vi "Waveform.vi"() -> ()   [LabVIEW 2016]
uses:
  controls/ScanWaveform.ctl
  controls/Enum.ctl
  <vilib>/Utility/error.llb/Error Cluster From Error Code.vi
  <vilib>/rvi/errors/niLvFpgaAdjustHostInterfaceError.vi
  <vilib>/rvi/interface/nirviReadWriteControl/nirviReadWriteControl.xnode
  controls/FPGAVIreferenceTypeDefScanEngine.ctl
  FPGA Bitfiles/qnmController797_usbRIO_controllerFPGAmu_11012018-14h.lvbitx
  NiFpgaLv.dll
panel:
  in  "scanWaveFormCtl":T2={"slowWavePts"=1024, "fastWavePts"=1024, "slowWaveType"=enum."Triangle", "fastWaveType"=enum."Rounded", "slowRoundPts"=8, "fastRoundPts"=32, "Update Parameters"=FALSE, "Correct Hysteresis"=FALSE, "UpdateFPGA"=FALSE, "Update Graph"=FALSE, "Hysteresis comp?"=FALSE}
  out "Waveforms":waveform(dbl)[](graph)
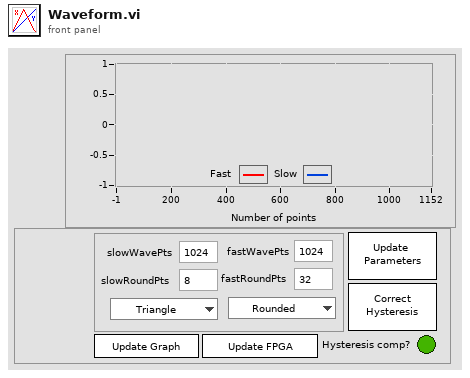
[diagram p1: front panel]
types:
  T1 = typedef "ScanWaveform.ctl" = enum16{"Sine", "Triangle", "Rounded"}
  T2 = cluster{"slowWavePts":u16, "fastWavePts":u16, "slowWaveType":T1, "fastWaveType":T1, "slowRoundPts":u16, "fastRoundPts":u16, "Update Parameters":bool, "Correct Hysteresis":bool, "UpdateFPGA":bool, "Update Graph":bool, "Hysteresis comp?":bool}
  T3 = enum16{"Init", "Update.Parameters", "Correct.Hysteresis", "Send.Waveform", "Refresh.Graph", "WaitForEvents", "Close"}
  T4 = typedef "Enum.ctl" = enum16{"Init", "Read", "Write"}
  T5 = cluster{"write":bool, "index":u16, "data":fxp<+/-,18,5>}
  T6 = cluster{"CorrectionToFGV":bool, "PolynomCoeff":dbl[], "CorrectionToFPGA":bool}
  T7 = typedef "FPGAVIreferenceTypeDefScanEngine.ctl" = refnum<k20>
  T8 = cluster{"slowWavePts":u16, "fastWavePts":u16, "slowWaveType":T1, "fastWaveType":T1, "slowRoundPts":u16, "fastRoundPts":u16, "singleDirectionScan":bool}
  T9 = cluster{"startFwd":u16, "endFwd":u16, "startBwd":u16, "endBwd":u16, "disableBlanking":bool, "useFineCounter":bool}
  T10 = cluster{"outputRate":u16, "fastDecFactor":u16, "outWaveSizeFast":u16, "pplUpsampling":u16, "numLines":u16, "se.p.fastInvDec":fxp<+,22,0>, "se.p.slowUpStep":fxp<+,28,0>, "se.p.outWaveSizeSlow":u16, "blankingMax":u32, "se.p.fastBlanking":cluster{"startFwd":u32, "endFwd":u32, "startBwd":u32, "endBwd":u32, "disableBlanking":bool, "useCoarseCounter":bool}}
  T11 = cluster{"Waveform Shape Fast In":dbl[], "Waveform Shape Slow In":dbl[]}
  T12 = cluster{"se.p.enable":bool, "se.p.singleDirection":bool, "se.p.haltScan":bool, "se.mot.p.start":bool}
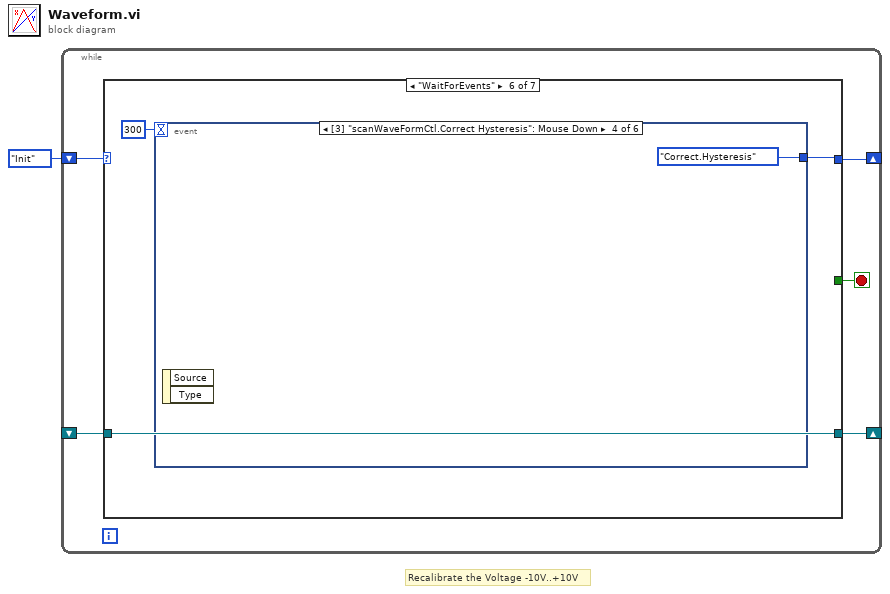
[diagram p0: block diagram]
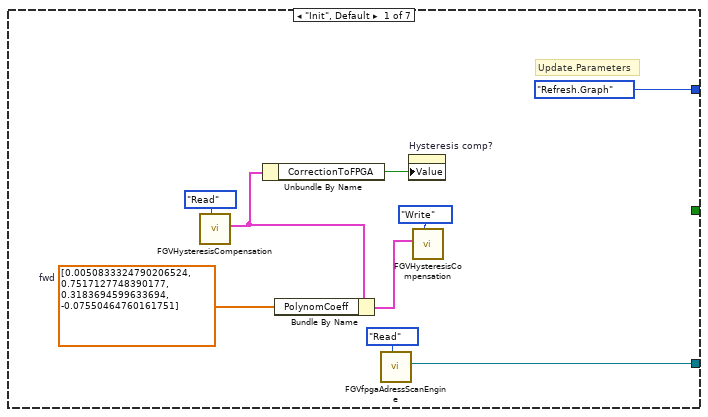
[diagram p2: hidden frame]
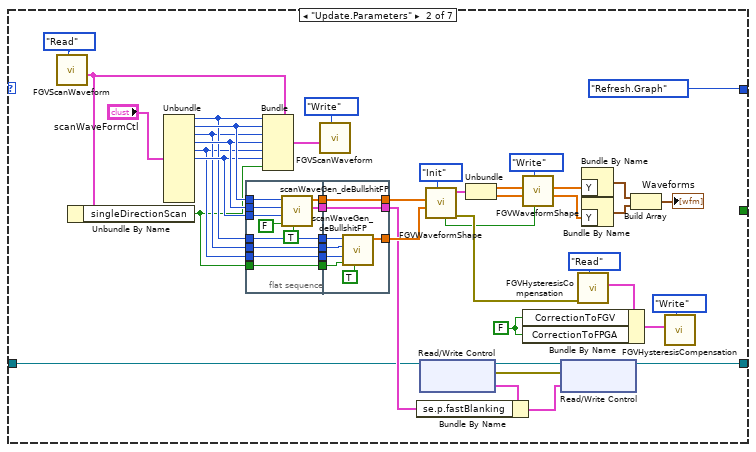
[diagram p3: hidden frame]
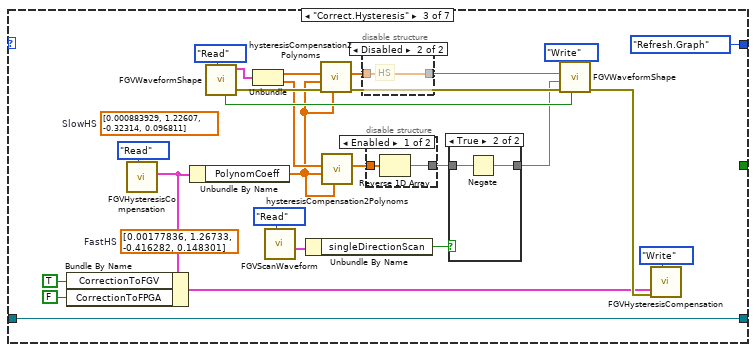
[diagram p4: hidden frame]
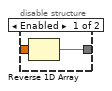
[diagram p5: hidden frame]
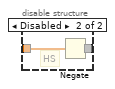
[diagram p6: hidden frame]
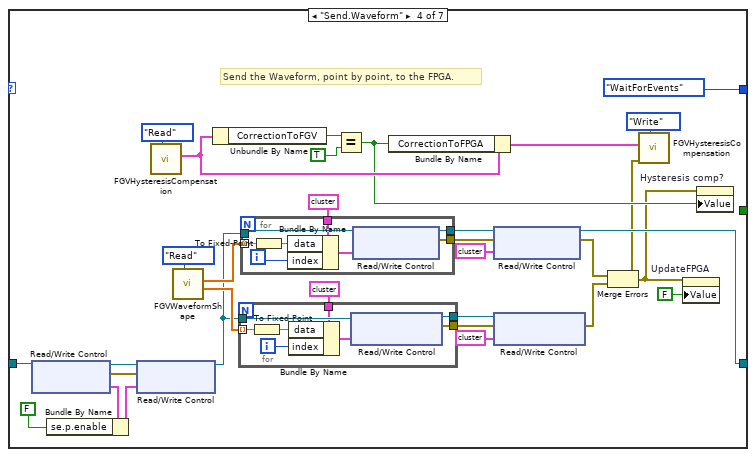
[diagram p8: hidden frame]
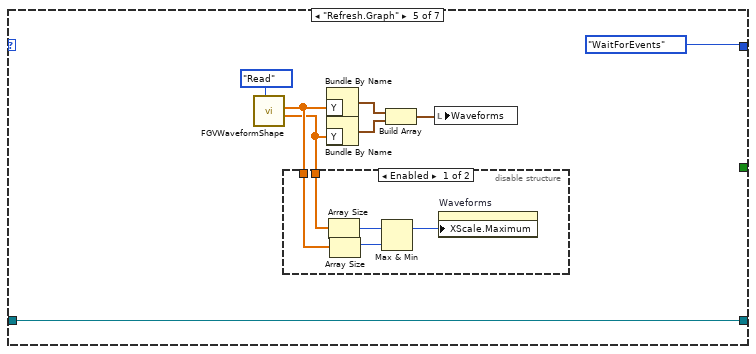
[diagram p9: hidden frame]
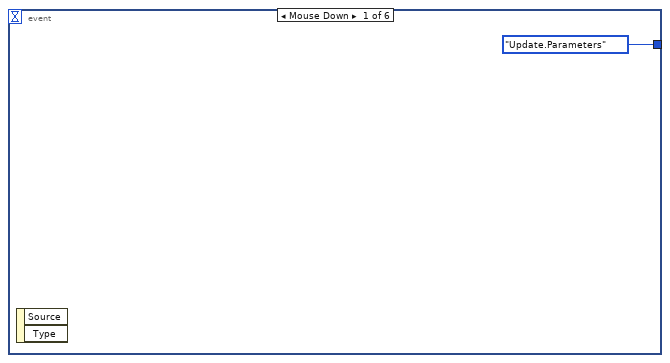
[diagram p11: hidden frame]
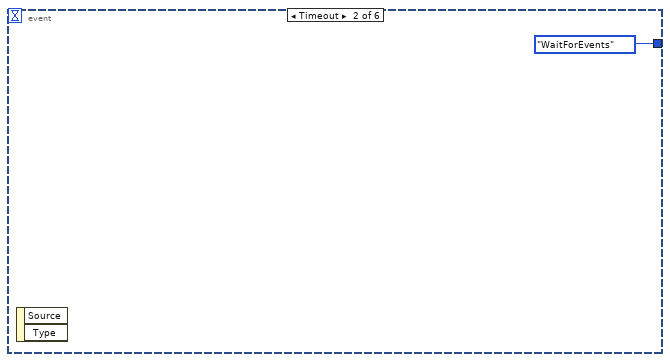
[diagram p12: hidden frame]
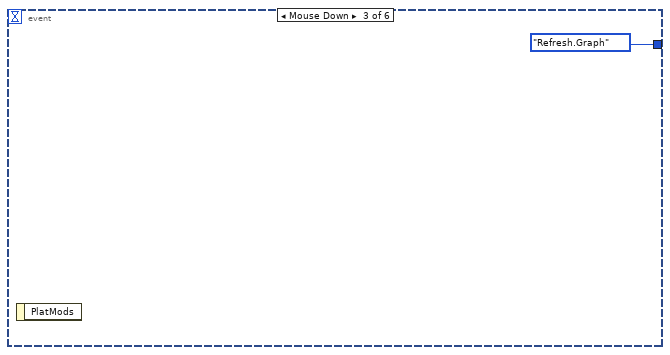
[diagram p13: hidden frame]
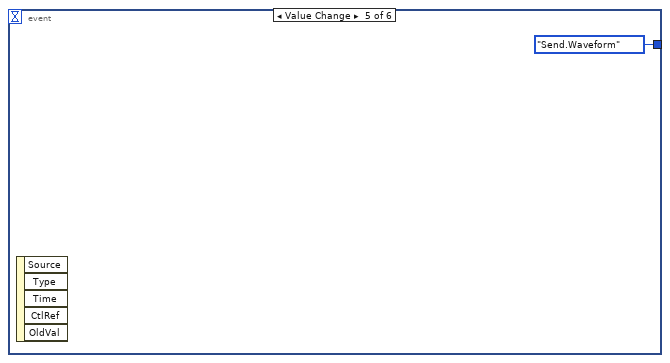
[diagram p14: hidden frame]
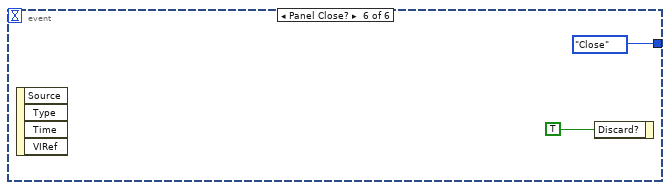
[diagram p15: hidden frame]
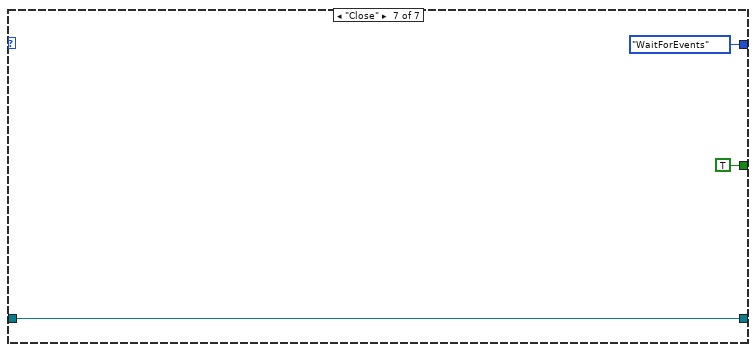
[diagram p16: hidden frame]
diagram:
  # "Recalibrate the Voltage -10V..+10V"
  n1 = while {
    shift-right: [w4] -> _
    shift-left: T3."Init" -> [w5]
    shift-right: [w3] -> _
    shift-left: _ -> [w2]
    stop <- w6 stop-if-true
    n2 = case shown="\"WaitForEvents\"" w5 {
      tunnel: [_ _ _ _ _ _ TRUE ("Discard?")] -> w6
      tunnel: [T3."Refresh.Graph" T3."Refresh.Graph" T3."Refresh.Graph" T3."WaitForEvents" T3."WaitForEvents" w177 T3."WaitForEvents"] -> w4
      tunnel: [w13 w32 w91 w126 w164 w176 w185] -> w3
      tunnel: w2 -> [_ w33 w91 w127 w164 w176 w185]
      frame "Init", Default {
        w7 = dbl[] [0.0050833324790206524, 0.7517127748390177, 0.3183694599633694, -0.07550464760161751]  # fwd
        # "Update.Parameters"
        n3 = call "FGVHysteresisCompensation.vi"("Enum"=Enum."Read") -> ("HysteresisOut"=w9:T6)  [unwired: 9 in, 1 out]
        n4 = Unbundle By Name(w9) -> ("CorrectionToFPGA"=w8:bool)
        n5 = Bundle By Name(cluster=w9, "PolynomCoeff"=w7) -> (w10:T6)
        n6 = call "FGVfpgaAdressScanEngine.vi"("Enum"=Enum."Read") -> ("FPGA.SEout"=w13:T7)  [unwired: 6 in, 4 out]
        n7 = property on="Hysteresis comp?" class="Bool (strict)"("Value"=w8) -> ()  [unwired: 2 in, 2 out]
        n8 = call "FGVHysteresisCompensation.vi"("Enum"=Enum."Write", "HysteresisIn"=w10) -> ()  [unwired: 8 in, 2 out]
      }
      frame "Update.Parameters" {
        w26 = FALSE ("Correction?")
        n9 = call "FGVScanWaveform.vi"("Enum"=Enum."Read") -> ("scanWaveFormCtl Out"=w45:T8)  [unwired: 9 in, 1 out]
        n10 = Unbundle By Name(w45) -> ("singleDirectionScan"=w38:bool)
        n11 = Unbundle("scanWaveFormCtl") -> ("slowWavePts"=w41:u16, "fastWavePts"=w44:u16, "slowWaveType"=w40:T1, "fastWaveType"=w43:T1, "slowRoundPts"=w39:u16, "fastRoundPts"=w42:u16)  [unwired: 5 out]
        n12 = flat-sequence {
          tunnel: w44 -> [w70]
          tunnel: w43 -> [w69]
          tunnel: w42 -> [w68]
          tunnel: [w66] -> w59
          tunnel: w41 -> [w66]
          tunnel: w40 -> [w65]
          tunnel: [w65] -> w58
          tunnel: [w64] -> w57
          tunnel: w39 -> [w64]
          tunnel: w38 -> [w63]
          tunnel: [w63] -> w56
          tunnel: [w62] -> w55
          tunnel: [w61] -> w54
          tunnel: w59 -> [w73]
          tunnel: w58 -> [w78]
          tunnel: w57 -> [w77]
          tunnel: w56 -> [w76]
          tunnel: w55 -> [w75]
          tunnel: [w75] -> w37
          tunnel: [w74] -> w36
          tunnel: w54 -> [w72]
          tunnel: [w72] -> w35
          frame #0 {
            n13 = call "scanWaveGen_deBullshitFP.vi"("overScanBlanking"=TRUE, "singleDirScan"=FALSE, "numRoundingPts"=w68, "scanWaveForm"=w69, "numPts"=w70) -> ("blankingParams"=w61:T9, "outWave"=w62:dbl[])  [unwired: 5 in]
          }
          frame #1 {
            n14 = call "scanWaveGen_deBullshitFP.vi"("overScanBlanking"=TRUE, "singleDirScan"=w76, "numRoundingPts"=w77, "scanWaveForm"=w78, "numPts"=w73) -> ("outWave"=w74:dbl[])  [unwired: 5 in, 1 out]
          }
        }
        n15 = Bundle(cluster=w45, "slowWavePts"=w41, "fastWavePts"=w44, "slowWaveType"=w40, "fastWaveType"=w43, "slowRoundPts"=w39, "fastRoundPts"=w42, "singleDirectionScan"=w38) -> (w47:T8)
        n16 = call "FGVScanWaveform.vi"("Enum"=Enum."Write", "scanWaveFormCtl In"=w47) -> ()  [unwired: 8 in, 2 out]
        n17 = xnode "Read/Write Control"("FPGA VI Reference In"=w33) -> ("error out"=w24:errorcluster, "se.p.clocks"=w23:T10)  [unwired: 1 in, 1 out]
        n18 = Bundle By Name(cluster=w23, "se.p.fastBlanking"=w35) -> (w22:T10)
        n19 = call "FGVWaveformShape.vi"("Enum"=Enum."Init", "Waveform Shape Slow In"=w36, "Waveform Shape Fast In"=w37) -> ("error out"=w25:errorcluster, "WaveformInit"=w31:T11, "Framing up? (down: f)"=w16:bool)  [unwired: 4 in, 2 out]
        n20 = Unbundle(w31) -> ("Waveform Shape Fast In"=w20:dbl[], "Waveform Shape Slow In"=w18:dbl[])
        n21 = call "FGVWaveformShape.vi"("Framing up? (down: f)"=w16, "Enum"=Enum."Write", "Waveform Shape Slow In"=w18, "Waveform Shape Fast In"=w20) -> ("Waveform Shape Slow Out"=w17:dbl[], "Waveform Shape Fast Out"=w19:dbl[])  [unwired: 3 in, 3 out]
        n22 = xnode "Read/Write Control"("FPGA VI Reference In"=w33, "error in"=w24, "se.p.clocks"=w22) -> ("FPGA VI Reference Out"=w32:T7)  [unwired: 1 out]
        n23 = call "FGVHysteresisCompensation.vi"("Enum"=Enum."Read", "error in"=w25) -> ("HysteresisOut"=w28:T6)  [unwired: 8 in, 1 out]
        n24 = Bundle By Name(cluster=w28, "CorrectionToFGV"=w26, "CorrectionToFPGA"=w26) -> (w27:T6)
        n25 = Bundle By Name("Y"=w19) -> (w51:waveform(dbl))  [unwired: 1 in]
        n26 = Bundle By Name("Y"=w17) -> (w52:waveform(dbl))  [unwired: 1 in]
        n27 = Build Array(w51, w52) -> (→"Waveforms":waveform(dbl)[])
        n28 = call "FGVHysteresisCompensation.vi"("Enum"=Enum."Write", "HysteresisIn"=w27) -> ()  [unwired: 8 in, 2 out]
      }
      frame "Correct.Hysteresis" {
        (unwired) dbl[] [0.00177836, 1.26733, -0.416282, 0.148301]  # FastHS
        (unwired) dbl[] [0.000883929, 1.22607, -0.32314, 0.096811]  # SlowHS
        n29 = call "FGVHysteresisCompensation.vi"("Enum"=Enum."Read") -> ("HysteresisOut"=w86:T6)  [unwired: 9 in, 1 out]
        n30 = Bundle By Name(cluster=w86, "CorrectionToFGV"=TRUE ("Correction?"), "CorrectionToFPGA"=FALSE) -> (w87:T6)
        n31 = Unbundle By Name(w86) -> ("PolynomCoeff"=w79:dbl[])
        n32 = call "FGVWaveformShape.vi"("Enum"=Enum."Read") -> ("error out"=w95:errorcluster, "WaveformInit"=w96:T11, "Framing up? (down: f)"=w98:bool)  [unwired: 6 in, 2 out]
        n33 = Unbundle(w96) -> ("Waveform Shape Fast In"=w100:dbl[], "Waveform Shape Slow In"=w94:dbl[])
        n34 = call "FGVScanWaveform.vi"("Enum"=Enum."Read") -> ("scanWaveFormCtl Out"=w82:T8)  [unwired: 9 in, 1 out]
        n35 = Unbundle By Name(w82) -> ("singleDirectionScan"=w80:bool)
        n36 = call "hysteresisCompensation2Polynoms.vi"("PolynomBWD"=w79, "error in (no error)"=w95, "PolynomFWD"=w79, "Uncorrected Shape"=w100) -> ("error out"=w103:errorcluster, "Corrected Shape"=w99:dbl[])  [unwired: 6 in]
        n37 = call "hysteresisCompensation2Polynoms.vi"("PolynomBWD"=w79, "PolynomFWD"=w79, "Uncorrected Shape"=w94) -> ("Corrected Shape"=w93:dbl[])  [unwired: 7 in, 1 out]
        n38 = disable-structure shown="Disabled" {
          disable-tunnel: [w106 w107] -> w101
          disable-tunnel: w99 -> [w105 w107]
          frame Enabled {
            n39 = Reverse 1D Array(array=w105) -> (reversed array=w106:dbl[])
          }
          frame Disabled {
            # "HS"
          }
        }
        n40 = disable-structure shown="Enabled" {
          disable-tunnel: w93 -> [w109 w111]
          disable-tunnel: [w108 w110] -> w81
          frame Enabled {
            n41 = Reverse 1D Array(array=w109) -> (reversed array=w108:dbl[])
          }
          frame Disabled {
            # "HS"
            n42 = Negate(x=w111) -> (-x=w110:dbl[])
          }
        }
        n43 = case shown="True" w80 {
          tunnel: [w112 w114] -> w90
          tunnel: w81 -> [w112 w113]
          frame False {
          }
          frame True {
            n44 = Negate(x=w113) -> (-x=w114:dbl[])
          }
        }
        n45 = call "FGVWaveformShape.vi"("Framing up? (down: f)"=w98, "Enum"=Enum."Write", "error in"=w103, "Waveform Shape Slow In"=w90, "Waveform Shape Fast In"=w101) -> ("error out"=w104:errorcluster)  [unwired: 2 in, 4 out]
        n46 = call "FGVHysteresisCompensation.vi"("Enum"=Enum."Write", "error in"=w104, "HysteresisIn"=w87) -> ()  [unwired: 7 in, 2 out]
      }
      frame "Send.Waveform" {
        # "Send the Waveform, point by point, to the FPGA."
        n47 = xnode "Read/Write Control"("FPGA VI Reference In"=w127) -> ("FPGA VI Reference Out"=w137:T7, "error out"=w138:errorcluster, "se.p.modes"=w139:T12)  [unwired: 1 in]
        n48 = Bundle By Name(cluster=w139, "se.p.enable"=FALSE ("scanEnabled")) -> (w141:T12)
        n49 = xnode "Read/Write Control"("FPGA VI Reference In"=w137, "error in"=w138, "se.p.modes"=w141) -> ("FPGA VI Reference Out"=w140:T7)  [unwired: 1 out]
        n50 = call "FGVHysteresisCompensation.vi"("Enum"=Enum."Read") -> ("HysteresisOut"=w118:T6)  [unwired: 9 in, 1 out]
        n51 = call "FGVWaveformShape.vi"("Enum"=Enum."Read") -> ("Waveform Shape Slow Out"=w145:dbl[], "Waveform Shape Fast Out"=w144:dbl[])  [unwired: 6 in, 3 out]
        n52 = Unbundle By Name(w118) -> ("CorrectionToFGV"=w120:bool)
        n53 = for {
          tunnel: [w152] -> w134
          tunnel: w145 -> [w151] mode=indexing
          tunnel: T5 {"write"=TRUE, "index"=0, "data"=0.0} ("slowWaveWrite") -> [w147]
          tunnel: w140 -> [w150]
          tunnel: [w153] -> w133
          i -> [w146]
          n54 = To Fixed-Point(number=w151) -> (fixed-point=w148:fxp<+/-,18,5>)  [unwired: 1 in]
          n55 = Bundle By Name(cluster=w147, "data"=w148, "index"=w146) -> (w149:T5)
          n56 = xnode "Read/Write Control"("FPGA VI Reference In"=w150, "se.m.slowAxis"=w149) -> ("FPGA VI Reference Out"=w153:T7, "error out"=w152:errorcluster)  [unwired: 1 in]
        }
        n57 = for {
          tunnel: [w160] -> w131
          tunnel: w144 -> [w159] mode=indexing
          tunnel: T5 {"write"=TRUE, "index"=0, "data"=0.0} ("slowWaveWrite") -> [w155]
          tunnel: w140 -> [w158]
          tunnel: [w161] -> w130
          i -> [w154]
          n58 = To Fixed-Point(number=w159) -> (fixed-point=w156:fxp<+/-,18,5>)  [unwired: 1 in]
          n59 = Bundle By Name(cluster=w155, "data"=w156, "index"=w154) -> (w157:T5)
          n60 = xnode "Read/Write Control"("FPGA VI Reference In"=w158, "se.m.fastAxis"=w157) -> ("FPGA VI Reference Out"=w161:T7, "error out"=w160:errorcluster)  [unwired: 1 in]
        }
        n61 = Equal?(x=w120, y=TRUE) -> (x = y?=w116:bool)
        n62 = Bundle By Name(cluster=w118, "CorrectionToFPGA"=w116) -> (w117:T6)
        n63 = xnode "Read/Write Control"("FPGA VI Reference In"=w130, "error in"=w131, "se.m.fastAxis"=T5 {"write"=FALSE, "index"=0, "data"=0.0} ("fastWaveWrite")) -> ("FPGA VI Reference Out"=w126:T7, "error out"=w125:errorcluster)
        n64 = xnode "Read/Write Control"("FPGA VI Reference In"=w133, "error in"=w134, "se.m.slowAxis"=T5 {"write"=FALSE, "index"=0, "data"=0.0} ("fastWaveWrite")) -> ("error out"=w124:errorcluster)  [unwired: 1 out]
        n65 = Merge Errors(w125, w124) -> (w115:errorcluster)
        n66 = call "FGVHysteresisCompensation.vi"("Enum"=Enum."Write", "error in"=w115, "HysteresisIn"=w117) -> ()  [unwired: 7 in, 2 out]
        n67 = property on="UpdateFPGA" class="Bool (strict)"(error in=w115, "Value"=FALSE) -> ()  [unwired: 1 in, 2 out]
        n68 = property on="Hysteresis comp?" class="Bool (strict)"(error in=w115, "Value"=w116) -> ()  [unwired: 1 in, 2 out]
      }
      frame "Refresh.Graph" {
        n69 = call "FGVWaveformShape.vi"("Enum"=Enum."Read") -> ("Waveform Shape Slow Out"=w162:dbl[], "Waveform Shape Fast Out"=w163:dbl[])  [unwired: 6 in, 3 out]
        n70 = disable-structure shown="Enabled" {
          disable-tunnel: w163 -> [w174 _]
          disable-tunnel: w162 -> [w173 _]
          frame Enabled {
            n71 = Array Size(array=w173) -> (size(s)=w172:i32)
            n72 = Array Size(array=w174) -> (size(s)=w171:i32)
            n73 = Max & Min(x=w172, y=w171) -> (max(x,y)=w170:i32)  [unwired: 1 out]
            n74 = property on="Waveforms" class="WFGraph (strict)"("XScale.Maximum"=w170) -> ()  [unwired: 2 in, 2 out]
          }
          frame Disabled {
          }
        }
        n75 = Bundle By Name("Y"=w163) -> (w167:waveform(dbl))  [unwired: 1 in]
        n76 = Bundle By Name("Y"=w162) -> (w168:waveform(dbl))  [unwired: 1 in]
        n77 = Build Array(w167, w168) -> (w169:waveform(dbl)[])
        n78 = local write "Waveforms"(w169) -> ()
      }
      frame "WaitForEvents" {
        n79 = event shown="[3] \"scanWaveFormCtl.Correct Hysteresis\": Mouse Down" {
          selector: _ -> [_ _ _ _ _ _]
          dyn-events: _ -> [_ _ _ _ _ _]
          timeout: 300 -> [_ _ _ _ _ _]
          tunnel: [T3."Update.Parameters" T3."WaitForEvents" T3."Refresh.Graph" T3."Correct.Hysteresis" T3."Send.Waveform" T3."Close"] -> w177
          event "scanWaveFormCtl.Update Parameters": Mouse Down {
            n80 = event-data() -> ()  [unwired: 1 in, 2 out]
          }
          event Timeout {
            n81 = event-data() -> ()  [unwired: 1 in, 2 out]
          }
          event "scanWaveFormCtl.Update Graph": Mouse Down {
            n82 = event-data() -> ()  [unwired: 1 in, 1 out]
          }
          event "scanWaveFormCtl.Correct Hysteresis": Mouse Down {
            n83 = event-data() -> ()  [unwired: 1 in, 2 out]
          }
          event "scanWaveFormCtl.UpdateFPGA": Value Change {
            n84 = event-data() -> ()  [unwired: 1 in, 5 out]
          }
          event Panel Close? {
            n85 = event-data() -> ()  [unwired: 1 in, 4 out]
            n86 = event-data("Discard?"=TRUE) -> ()  [unwired: 1 in, 1 out]
          }
        }
      }
      frame "Close" {
      }
    }
  }
